vi "GUI AIP.vi"(10 "AIP Status":T1, 11 "Cluster in":refnum<vi>) -> ()   [LabVIEW 2015, in "Shore Library.lvlib"]
uses:
  Shore Library.lvlib
  Libraries/RDS Instruments/AIP/AIP Status.ctl
  Libraries/RDS Instruments/AIP/AIP States.ctl
  Libraries/RDS Instruments/RDS Instrument Library.lvlib
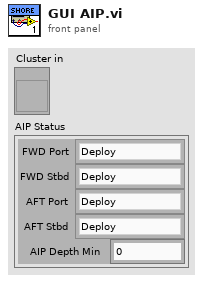
[diagram p1: front panel]
types:
  T1 = typedef "RDS Instrument Library.lvlib/AIP Status.ctl" = cluster{"FWD Port":T2, "FWD Stbd":T2, "AFT Port":T2, "AFT Stbd":T2, "AIP Depth Min":u8}
  T2 = typedef "RDS Instrument Library.lvlib/AIP States.ctl" = enum16{"Deploy", "Deploying", "Deployed", "Stow", "Stowing", "Stowed", "Fault", "brakeOnStow", "breakOnDeploy", "Stopped", "Stopping"}
  T3 = cluster{"FP":refnum<vi>, "FS":refnum<vi>, "AP":refnum<vi>, "AS":refnum<vi>}
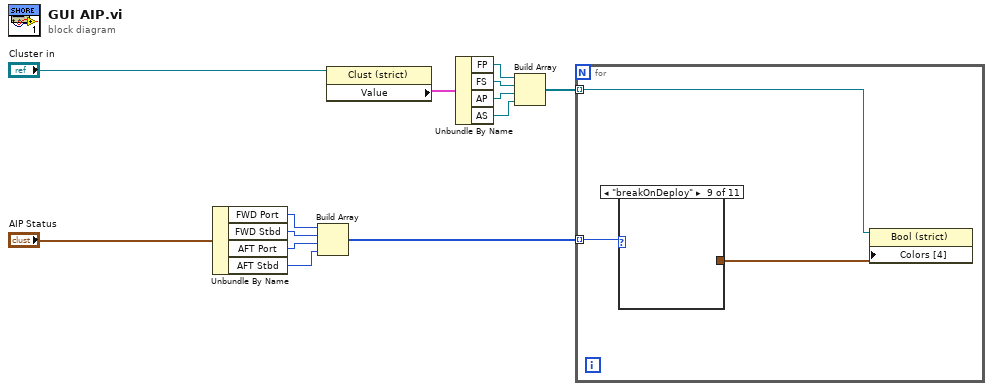
[diagram p0: block diagram]
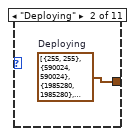
[diagram p3: hidden frame]
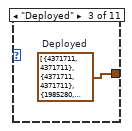
[diagram p4: hidden frame]
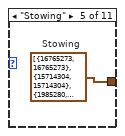
[diagram p6: hidden frame]
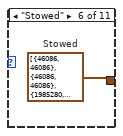
[diagram p7: hidden frame]
diagram:
  n1 = Unbundle By Name("AIP Status") -> ("FWD Port"=w5:T2, "FWD Stbd"=w4:T2, "AFT Port"=w3:T2, "AFT Stbd"=w2:T2)
  n2 = Build Array(w5, w4, w3, w2) -> (w1:T2[])
  n3 = property class="Clust (strict)"(reference="Cluster in") -> ("Value"=w11:T3)  [unwired: 1 in, 2 out]
  n4 = Unbundle By Name(w11) -> ("FP"=w10:refnum<vi>, "FS"=w9:refnum<vi>, "AP"=w8:refnum<vi>, "AS"=w7:refnum<vi>)
  n5 = Build Array(w10, w9, w8, w7) -> (w6:refnum<vi>[])
  n6 = for {
    tunnel: w6 -> [w16] mode=indexing
    tunnel: w1 -> [w15] mode=indexing
    n7 = case shown="\"breakOnDeploy\"" w15 {
      tunnel: [_ w17 w18 _ w19 w20 _ _ _ _ _] -> w14
      frame "Deploy", Default {
      }
      frame "Deploying" {
        w17 = cluster{u32, u32}[] [{255, 255}, {590024, 590024}, {1985280, 1985280}, {6618880, 6618880}]  # Deploying
      }
      frame "Deployed" {
        w18 = cluster{u32, u32}[] [{4371711, 4371711}, {4371711, 4371711}, {1985280, 1985280}, {6618880, 6618880}]  # Deployed
      }
      frame "Stow" {
      }
      frame "Stowing" {
        w19 = cluster{u32, u32}[] [{16765273, 16765273}, {15714304, 15714304}, {1985280, 1985280}, {6618880, 6618880}]  # Stowing
      }
      frame "Stowed" {
        w20 = cluster{u32, u32}[] [{46086, 46086}, {46086, 46086}, {1985280, 1985280}, {6618880, 6618880}]  # Stowed
      }
      frame "Fault" {
      }
      frame "brakeOnStow" {
      }
      frame "breakOnDeploy" {
      }
      frame "Stopped" {
      }
      frame "Stopping" {
      }
    }
    n8 = property class="Bool (strict)"(reference=w16, "Colors [4]"=w14) -> ()  [unwired: 1 in, 2 out]
  }
